vi "Find_Mirror_Up_Down_Strings.vi"(2 "Filenames":string[](array[string])) -> (0 "Base Filenames to display":string[](array[string]), 1 "1st Basename":string)   [LabVIEW 2022 SP3]
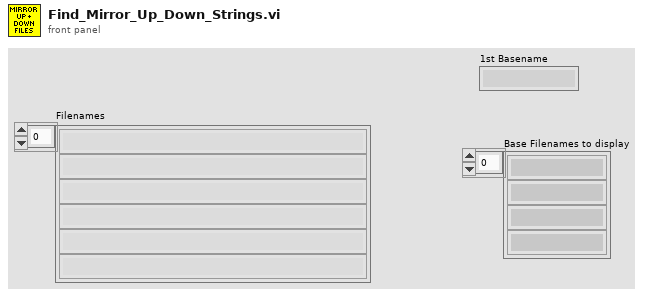
[diagram p1: front panel]
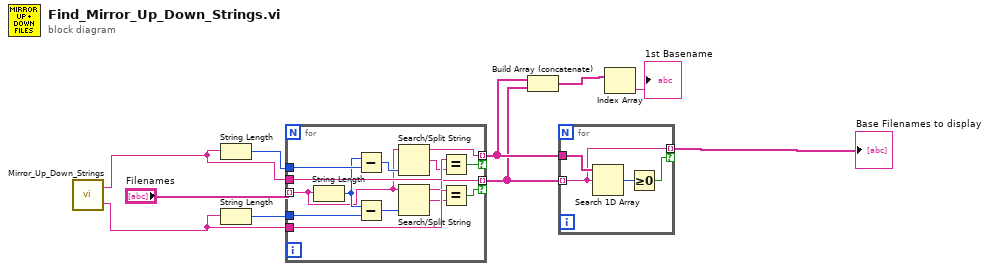
[diagram p0: block diagram]
diagram:
  n1 = call "Mirror_Up_Down_Strings.vi"() -> ("Mirror Down"=w8:string, "Mirror Up"=w9:string)  [unwired: 2 in]
  n2 = String Length(string=w9) -> (length=w6:i32)
  n3 = String Length(string=w8) -> (length=w5:i32)
  n4 = for {
    tunnel: "Filenames" -> [w16] mode=indexing
    tunnel: w6 -> [w22]
    tunnel: w9 -> [w24]
    tunnel: w5 -> [w18]
    tunnel: w8 -> [w23]
    tunnel: [w14] -> w3 mode=indexing if=w13
    tunnel: [w12] -> w4 mode=indexing if=w11
    n5 = String Length(string=w16) -> (length=w19:i32)
    n6 = Subtract(x=w19, y=w22) -> (x-y=w21:i32)
    n7 = Subtract(x=w19, y=w18) -> (x-y=w17:i32)
    n8 = Search/Split String(string=w16, offset (0)=w21) -> (substring before match=w12:string, match + rest of string=w20:string)  [unwired: 1 in, 1 out]
    n9 = Search/Split String(string=w16, offset (0)=w17) -> (substring before match=w14:string, match + rest of string=w15:string)  [unwired: 1 in, 1 out]
    n10 = Equal?(x=w24, y=w20) -> (x = y?=w11:bool)
    n11 = Equal?(x=w23, y=w15) -> (x = y?=w13:bool)
  }
  n12 = Build Array (concatenate)(w4, w3) -> (w2:string[])
  n13 = for {
    tunnel: w4 -> [w28]
    tunnel: w3 -> [w26] mode=indexing
    tunnel: [w26] -> w7 mode=indexing if=w25
    n14 = Search 1D Array(1D array=w28, element=w26) -> (index of element=w27:i32)  [unwired: 1 in]
    n15 = Greater Or Equal To 0?(x=w27) -> (x >= 0?=w25:bool)
  }
  "Base Filenames to display" <- w7
  n16 = Index Array(array=w2) -> (element=→"1st Basename":string)  [unwired: 1 in]
